vi "host_with_subvis.vi"() -> ()   [LabVIEW 2014]
uses:
  <vilib>/userdefined/High Color/nirio_resource_hc.ctl
  <instrlib>/niSync/niSync.llb/niSync Initialize (IVI).vi
  <vilib>/FPGAPlugInAG/Dynamic/niLvFpga_Close_Dynamic.vi
  <vilib>/rvi/interface/nirviCloseFPGA/nirviCloseFPGA.xnode
panel:
  in  "trigger  delay":u64
  in  "destination terminal":string(combo)="PXI_Trig0"
  out "Waveform Graph":waveform(dbl)(graph)
  out "Interleaved Raw Data":u64[](array[numeric])
  out "Counts":i16[][](array[numeric])
  out "Voltage":dbl[][](array[numeric])
  in  "num samples":u64=1000
  in  "FPGA name":T1 caption="RIO Device"
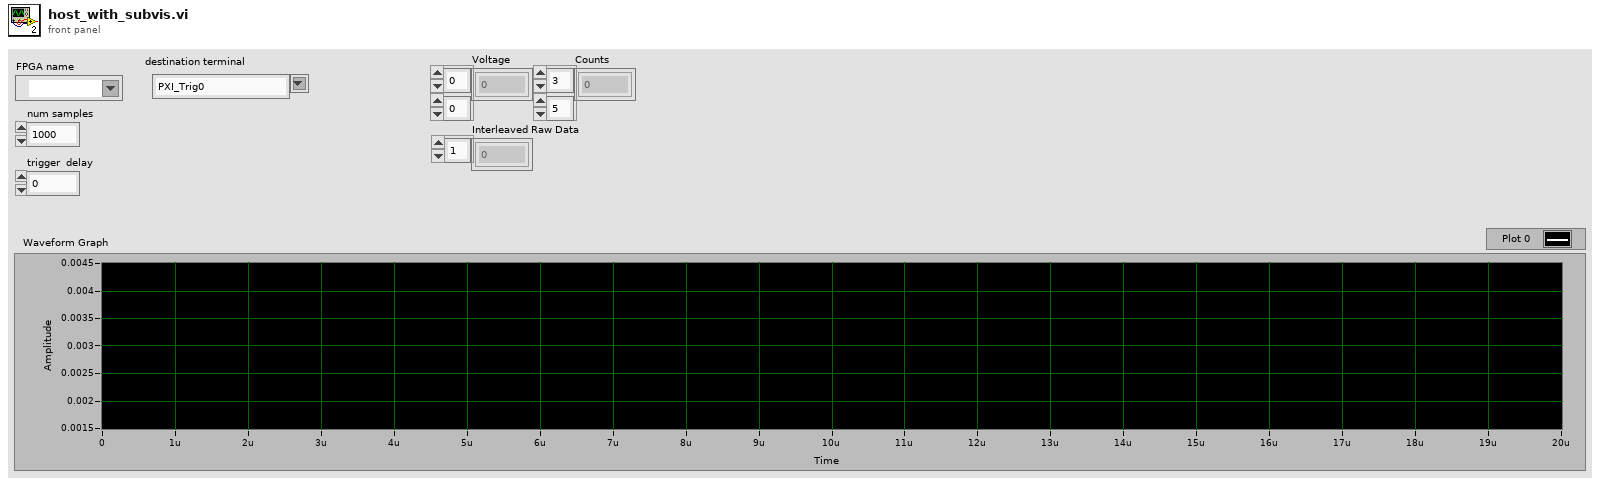
[diagram p1: front panel]
types:
  T1 = typedef "nirio_resource_hc.ctl" = tag
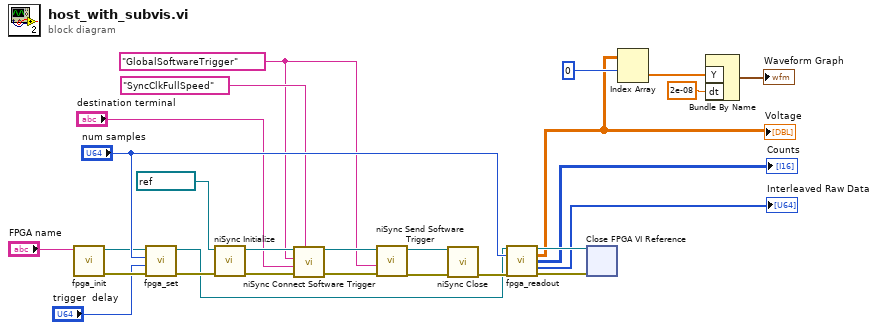
[diagram p0: block diagram]
diagram:
  w11 = "GlobalSoftwareTrigger" ("source terminal")
  n1 = call "fpga_init.vi"("FPGA name"="FPGA name") -> ("error out"=w27:errorcluster, "FPGA VI Reference Out"=w13:refnum<k20>)  [unwired: 9 in]
  n2 = call "fpga_set.vi"("error in"=w27, "trigger  delay"="trigger  delay", "num samples"="num samples", "FPGA VI Reference In"=w13) -> ("error out"=w18:errorcluster, "FPGA VI Reference Out"=w8:refnum<k20>)  [unwired: 6 in]
  n3 = call-poly <instrlib>:"niSync Initialize.vi"("error in (no error)"=w18, "resource name"=refnum<k15> "Sync0") -> ("error out"=w19:errorcluster, "instrument handle out"=w20:refnum<k15>)  [unwired: 8 in]
  n4 = call <instrlib>:"niSync Connect Software Trigger.vi"("synchronization clock"="SyncClkFullSpeed", "error in (no error)"=w19, "destination terminal"="destination terminal", "source terminal"=w11, "instrument handle"=w20) -> ("error out"=w21:errorcluster, "instrument handle out"=w22:refnum<k15>)  [unwired: 5 in]
  n5 = call <instrlib>:"niSync Send Software Trigger.vi"("error in (no error)"=w21, "source terminal"=w11, "instrument handle"=w22) -> ("error out"=w23:errorcluster, "instrument handle out"=w24:refnum<k15>)  [unwired: 7 in]
  n6 = call <instrlib>:"niSync Close.vi"("error in (no error)"=w23, "instrument handle"=w24) -> ("error out"=w17:errorcluster)  [unwired: 9 in]
  n7 = call "fpga_readout.vi"("FPGA VI Reference In"=w8, "samples"="num samples", "error in"=w17) -> ("FPGA Reference Out"=w4:refnum<k20>, "Voltage"=w1:dbl[][], "Counts"=→"Counts":i16[][], "Interleaved Raw Data"=→"Interleaved Raw Data":u64[], "error out"=w9:errorcluster)  [unwired: 8 in]
  "Voltage" <- w1
  n8 = xnode "Close FPGA VI Reference"("FPGA VI Reference In"=w4, "error in"=w9) -> ()  [unwired: 1 out]
  n9 = Index Array(array=w1, index (row)=0) -> (element=w6:dbl[])  [unwired: 1 in]
  n10 = Bundle By Name("Y"=w6, "dt"=2e-08) -> (→"Waveform Graph":waveform(dbl))  [unwired: 1 in]
